vi "PID_Calc.vi"(6 "Kd":dbl, 7 "dt":dbl=1.0 format="%0.2f", 9 "Error Signal":dbl format="%0.2f", 10 "Ki":dbl, 11 "Kp":dbl) -> (3 "PID Value":dbl)   [LabVIEW 2019]
uses:
  <vilib>/ptbypt/NI_PtbyPt.lvlib
panel:
  out "dx/dt":dbl format="%0.2f"
  out "integral x(t)":dbl format="%0.2f"
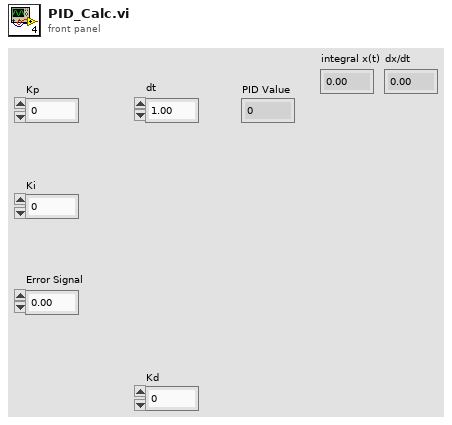
[diagram p1: front panel]
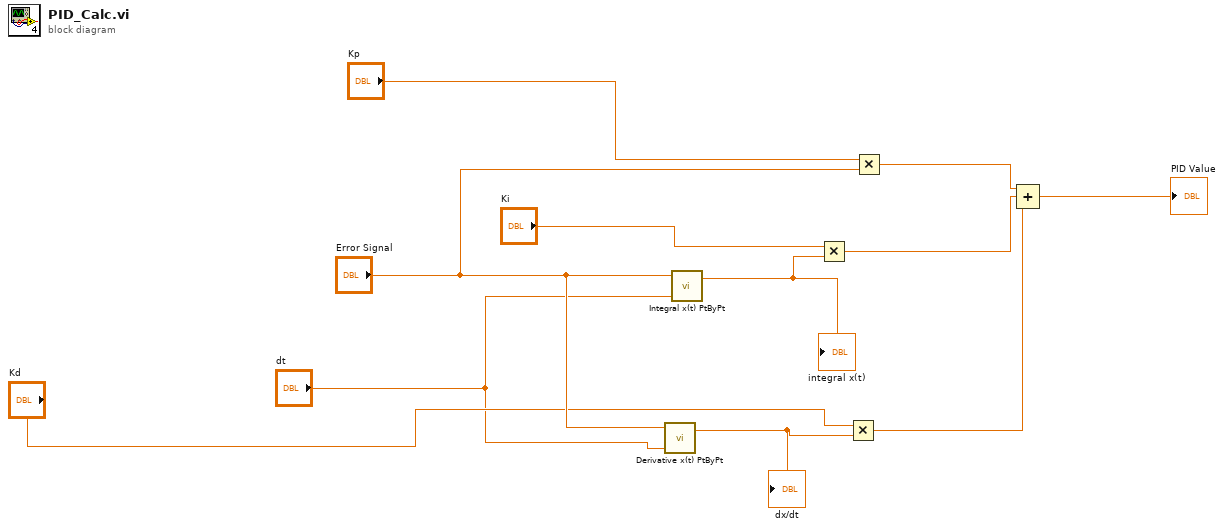
[diagram p0: block diagram]
diagram:
  n1 = call <vilib>:"Derivative x(t) PtByPt.vi"("dt"="dt", "x"="Error Signal") -> ("dx/dt"=w4:dbl)  [unwired: 2 in, 1 out]
  "dx/dt" <- w4
  n2 = call <vilib>:"Integral x(t) PtByPt.vi"("dt"="dt", "x"="Error Signal") -> ("integral x(t)"=w1:dbl)  [unwired: 2 in, 1 out]
  "integral x(t)" <- w1
  n3 = Multiply(x="Ki", y=w1) -> (x*y=w9:dbl)
  n4 = Multiply(x="Kd", y=w4) -> (x*y=w10:dbl)
  n5 = Multiply(x="Kp", y="Error Signal") -> (x*y=w8:dbl)
  n6 = Compound Arithmetic op=ADD(w8, w9, w10) -> (→"PID Value":dbl)
